vi "HRM-init-main.vi"(8 "error in (no error)":errorcluster) -> (0 "error out":errorcluster, 3 "init cluster":T1)   [LabVIEW 2020]
uses:
  HRM-init-cluster.ctl
  HRM-init-user_events.ctl
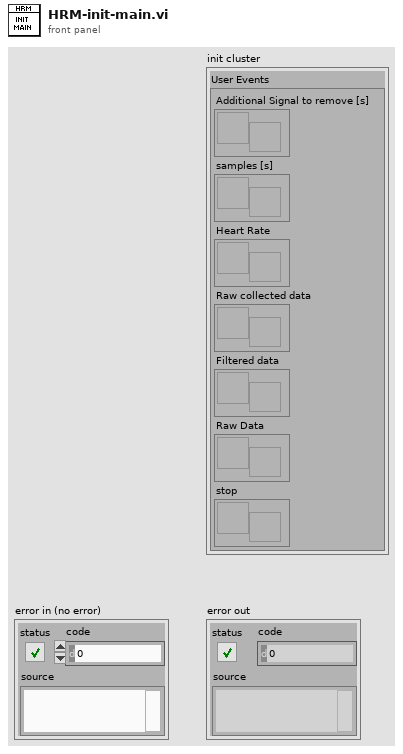
[diagram p1: front panel]
types:
  T1 = typedef "HRM-init-cluster.ctl" = cluster{"User Events":T2}
  T2 = typedef "HRM-init-user_events.ctl" = cluster{"Additional Signal to remove [s]":refnum<user-event>, "samples [s]":refnum<user-event>, "Heart Rate":refnum<user-event>, "Raw collected data":refnum<user-event>, "Filtered data":refnum<user-event>, "Raw Data":refnum<user-event>, "stop":refnum<user-event>}
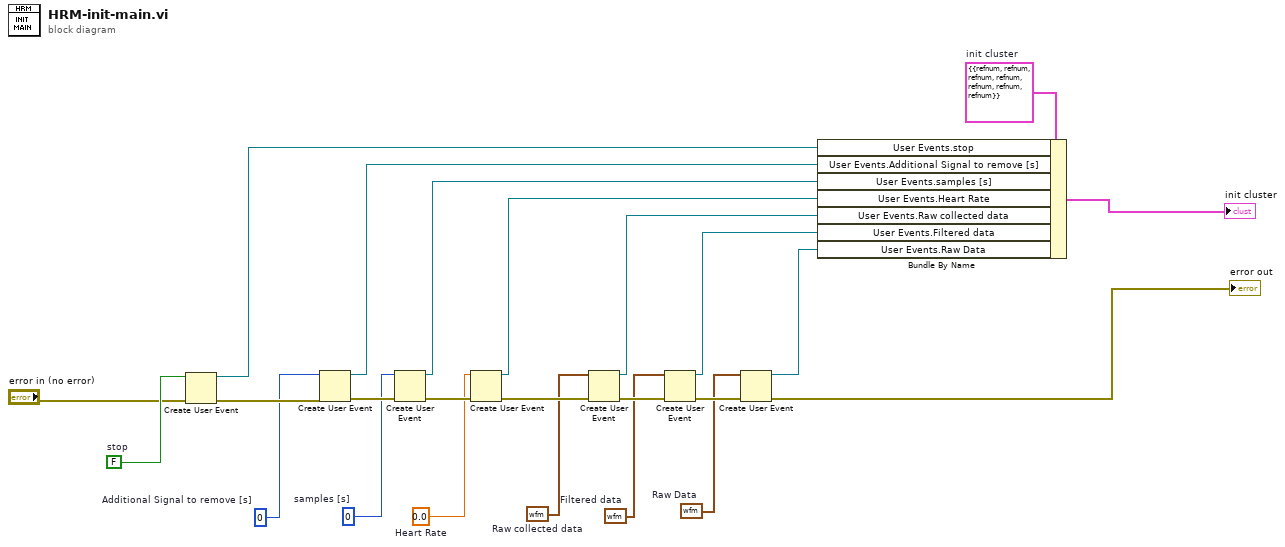
[diagram p0: block diagram]
diagram:
  w22 = FALSE  # stop
  w19 = T1 {"User Events"={"Additional Signal to remove [s]"=refnum, "samples [s]"=refnum, "Heart Rate"=refnum, "Raw collected data"=refnum, "Filtered data"=refnum, "Raw Data"=refnum, "stop"=refnum}}  # init cluster
  w4 = waveform(dbl) {"t0"=timestamp(0 s since 1904-01-01), "dt"=1.0, "Y"=[]}  # Raw collected data
  w3 = waveform(dbl) {"t0"=timestamp(0 s since 1904-01-01), "dt"=1.0, "Y"=[]}  # Filtered data
  w7 = 0  # samples [s]
  w6 = 0  # Additional Signal to remove [s]
  w5 = 0.0  # Heart Rate
  w1 = waveform(dbl) {"t0"=timestamp(0 s since 1904-01-01), "dt"=1.0, "Y"=[]}  # Raw Data
  n1 = Create User Event(user event datatype=w22, error in="error in (no error)") -> (user event=w23:refnum<user-event>, error out=w20:errorcluster)
  n2 = Create User Event(user event datatype=w6, error in=w20) -> (user event=w13:refnum<user-event>, error out=w14:errorcluster)
  n3 = Create User Event(user event datatype=w7, error in=w14) -> (user event=w12:refnum<user-event>, error out=w15:errorcluster)
  n4 = Create User Event(user event datatype=w5, error in=w15) -> (user event=w11:refnum<user-event>, error out=w16:errorcluster)
  n5 = Create User Event(user event datatype=w4, error in=w16) -> (user event=w10:refnum<user-event>, error out=w17:errorcluster)
  n6 = Create User Event(user event datatype=w3, error in=w17) -> (user event=w9:refnum<user-event>, error out=w18:errorcluster)
  n7 = Create User Event(user event datatype=w1, error in=w18) -> (user event=w8:refnum<user-event>, error out=→"error out":errorcluster)
  n8 = Bundle By Name(cluster=w19, "User Events.stop"=w23, "User Events.Additional Signal to remove [s]"=w13, "User Events.samples [s]"=w12, "User Events.Heart Rate"=w11, "User Events.Raw collected data"=w10, "User Events.Filtered data"=w9, "User Events.Raw Data"=w8) -> (→"init cluster":T1)
